vi "selection début série2_SD.vi"(1 "DATA":dbl[](array[numeric])) -> (0 "résultat début série":dbl[](array[numeric]))   [LabVIEW 2015]
uses:
  dependecies/globalVarSD.vi
panel:
  out "Data":dbl[](graph)
  out "Res":dbl[](graph)
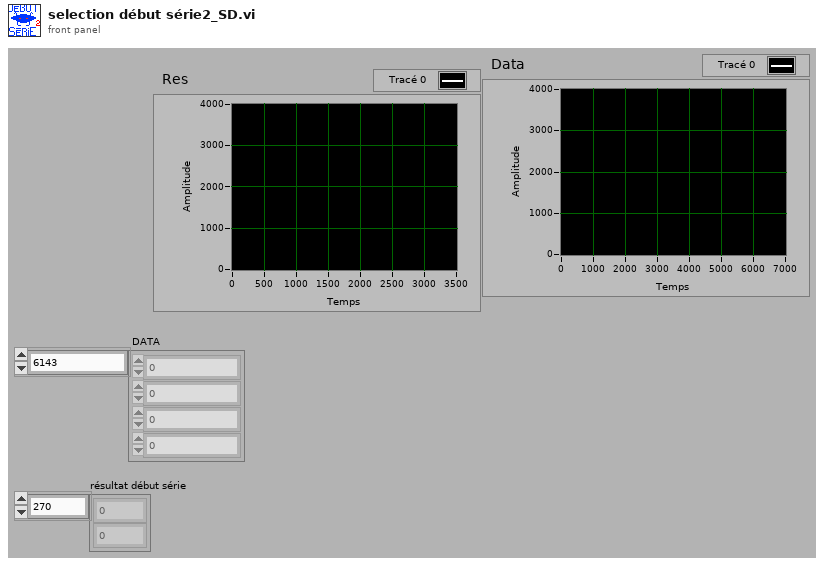
[diagram p1: front panel]
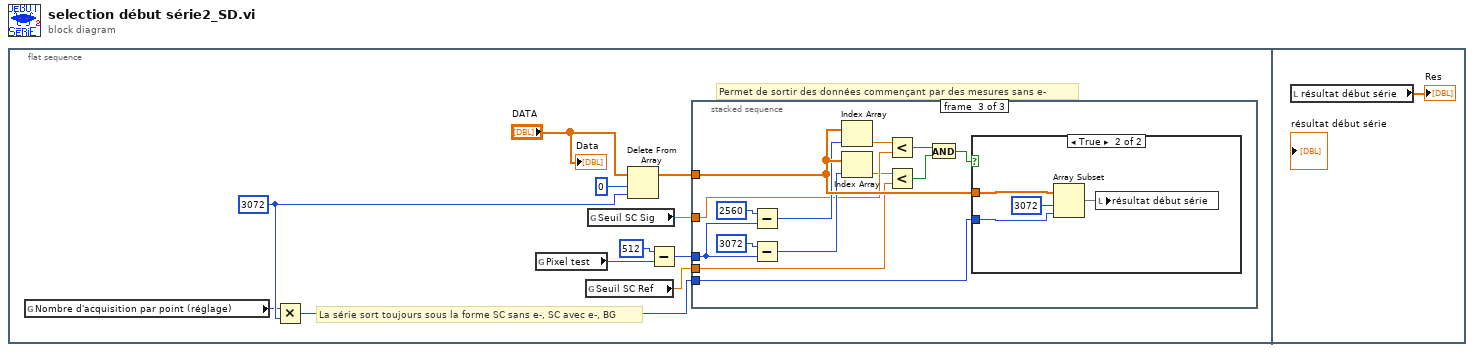
[diagram p0: block diagram]
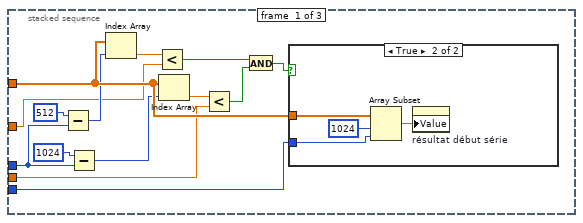
[diagram p2: hidden frame]
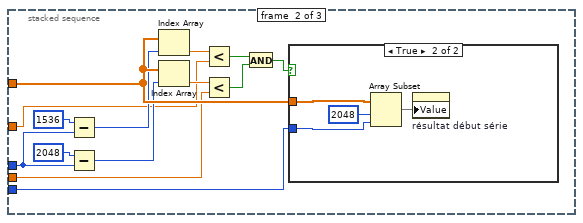
[diagram p4: hidden frame]
diagram:
  n1 = flat-sequence {
    frame #0 {
      w9 = 3072 ("y")
      # "Permet de sortir des données commençant par des mesures sans e-"
      # "La série sort toujours sous la forme SC sans e-, SC avec e-, BG"
      n2 = global read "globalVarSD.vi" "Nombre d'acquisition par point (réglage)"() -> (w5:u32)
      n3 = Multiply(x=w5, y=w9) -> (x*y=w11:u32)
      n4 = global read "globalVarSD.vi" "Pixel test"() -> (w6:u32)
      n5 = global read "globalVarSD.vi" "Seuil SC Ref"() -> (w4:dbl)
      n6 = global read "globalVarSD.vi" "Seuil SC Sig"() -> (w3:dbl)
      n7 = Delete From Array(array="DATA", length=0 ("longueur"), index=w9) -> (array with subset deleted=w1:dbl[])  [unwired: 1 out]
      n8 = Subtract(x=512 ("y"), y=w6) -> (x-y=w8:u32)
      n9 = stacked-sequence {
        tunnel: w11 -> [w21 w37 w58]
        tunnel: w1 -> [w20 w38 w57]
        tunnel: w8 -> [w18 w34 w53]
        tunnel: w3 -> [w13 w30 w50]
        tunnel: w4 -> [w12 w31 w48]
        frame #0 {
          n10 = Subtract(x=512 ("indice"), y=w18) -> (x-y=w15:u32)
          n11 = Subtract(x=1024 ("indice"), y=w18) -> (x-y=w14:u32)
          n12 = Index Array(array=w20, index=w15) -> (element=w25:dbl)
          n13 = Less?(x=w25, y=w13) -> (x < y?=w23:bool)
          n14 = Index Array(array=w20, index=w14) -> (element=w24:dbl)
          n15 = Less?(x=w24, y=w12) -> (x < y?=w22:bool)
          n16 = And(x=w23, y=w22) -> (x .and. y?=w19:bool)
          n17 = case shown="True" w19 {
            tunnel: w20 -> [_ w29]
            tunnel: w21 -> [_ w27]
            frame False {
            }
            frame True {
              n18 = Array Subset(array=w29, index=1024 ("indice"), length=w27) -> (w26:dbl[])
              n19 = property on="résultat début série" class="Arr (strict)"("Value"=w26) -> ()  [unwired: 2 in, 2 out]
            }
          }
        }
        frame #1 {
          n20 = Subtract(x=1536 ("indice"), y=w34) -> (x-y=w32:u32)
          n21 = Subtract(x=2048 ("indice"), y=w34) -> (x-y=w33:u32)
          n22 = Index Array(array=w38, index=w32) -> (element=w43:dbl)
          n23 = Index Array(array=w38, index=w33) -> (element=w42:dbl)
          n24 = Less?(x=w43, y=w30) -> (x < y?=w41:bool)
          n25 = Less?(x=w42, y=w31) -> (x < y?=w40:bool)
          n26 = And(x=w41, y=w40) -> (x .and. y?=w39:bool)
          n27 = case shown="True" w39 {
            tunnel: w37 -> [_ w46]
            tunnel: w38 -> [_ w45]
            frame False {
            }
            frame True {
              n28 = Array Subset(array=w45, index=2048 ("indice"), length=w46) -> (w44:dbl[])
              n29 = property on="résultat début série" class="Arr (strict)"("Value"=w44) -> ()  [unwired: 2 in, 2 out]
            }
          }
        }
        frame #2 {
          n30 = Subtract(x=2560 ("indice"), y=w53) -> (x-y=w54:u32)
          n31 = Subtract(x=3072 ("indice"), y=w53) -> (x-y=w51:u32)
          n32 = Index Array(array=w57, index=w54) -> (element=w61:dbl)
          n33 = Index Array(array=w57, index=w51) -> (element=w49:dbl)
          n34 = Less?(x=w61, y=w50) -> (x < y?=w60:bool)
          n35 = Less?(x=w49, y=w48) -> (x < y?=w59:bool)
          n36 = And(x=w60, y=w59) -> (x .and. y?=w56:bool)
          n37 = case shown="True" w56 {
            tunnel: w58 -> [_ w65]
            tunnel: w57 -> [_ w63]
            frame False {
            }
            frame True {
              n38 = Array Subset(array=w63, index=3072, length=w65) -> (w62:dbl[])
              n39 = local write "résultat début série"(w62) -> ()
            }
          }
        }
      }
      "Data" <- "DATA"
    }
    frame #1 {
      n40 = local read "résultat début série"() -> (→"Res":dbl[])
    }
  }
